vi "Get Section Names.vi"(8 "error in (no error)":errorcluster, 11 "Config in":refnum<class "LabVIEW-Config.lvclass">) -> (0 "error out":errorcluster, 1 "Section Names":string[](array[string]), 3 "Config out":refnum<class "LabVIEW-Config.lvclass">)   [LabVIEW 2017, in "LabVIEW-Config.lvlib" / "LabVIEW-Config.lvclass"]
uses:
  LabVIEW-Config.lvclass
  LabVIEW-Config.lvclass/LabVIEW-Config.ctl
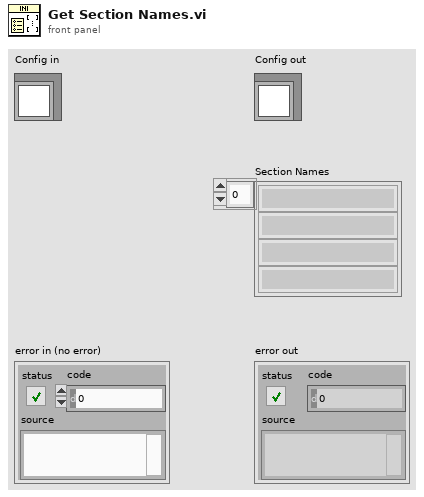
[diagram p1: front panel]
types:
  T1 = typedef "LabVIEW-Config.lvlib/LabVIEW-Config.lvclass/LineToken.ctl" = enum8{"comment", "section", "key", "more"}
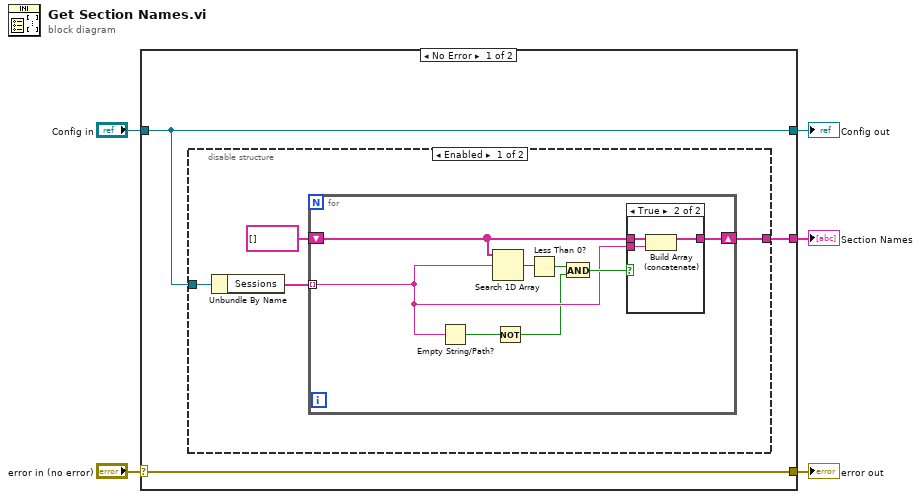
[diagram p0: block diagram]
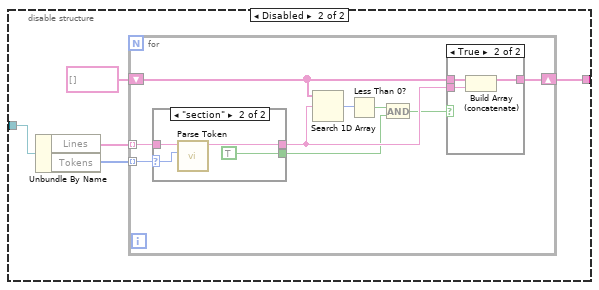
[diagram p3: hidden frame]
diagram:
  n1 = case shown="No Error" "error in (no error)" {
    selector: "error in (no error)" -> [w8 w48]
    tunnel: "Config in" -> [w7 w47]
    tunnel: [w6 _] -> w4
    tunnel: [w8 w48] -> w3
    tunnel: [w7 w47] -> w1
    frame No Error {
      n2 = disable-structure shown="Enabled" {
        disable-tunnel: w7 -> [w11 w27]
        disable-tunnel: [w9 w25] -> w6
        frame Enabled {
          n3 = Unbundle By Name(w11) -> ("Sessions"=w12:string[])
          n4 = for {
            tunnel: w12 -> [w15] mode=indexing
            shift-right: [w20] -> w9
            shift-left: string[] [] -> [w19]
            n5 = Empty String/Path?(string/path=w15) -> (empty?=w14:bool)
            n6 = Search 1D Array(1D array=w19, element=w15) -> (index of element=w18:i32)  [unwired: 1 in]
            n7 = Not(x=w14) -> (.not. x?=w13:bool)
            n8 = Less Than 0?(x=w18) -> (x < 0?=w17:bool)
            n9 = And(x=w17, y=w13) -> (x .and. y?=w16:bool)
            n10 = case shown="True" w16 {
              tunnel: [w21 w24] -> w20
              tunnel: w19 -> [w21 w23]
              tunnel: w15 -> [_ w22]
              frame False {
              }
              frame True {
                n11 = Build Array (concatenate)(w23, w22) -> (w24:string[])
              }
            }
          }
        }
        frame Disabled {
          n12 = Unbundle By Name(w27) -> ("Lines"=w28:string[], "Tokens"=w29:T1[])
          n13 = for {
            tunnel: w29 -> [w38] mode=indexing
            tunnel: w28 -> [w37] mode=indexing
            shift-right: [w36] -> w25
            shift-left: string[] [] -> [w35]
            n14 = case shown="\"section\"" w38 {
              selector: w38 -> [_ w44]
              tunnel: w37 -> [_ w45]
              tunnel: [_ w43] -> w34
              tunnel: [_ TRUE] -> w31
              frame Default {
              }
              frame "section" {
                n15 = call "Parse Token.vi"("Token"=w44, "Line"=w45) -> ("Name"=w43:string)  [unwired: 8 in, 1 out]
              }
            }
            n16 = Search 1D Array(1D array=w35, element=w34) -> (index of element=w33:i32)  [unwired: 1 in]
            n17 = Less Than 0?(x=w33) -> (x < 0?=w32:bool)
            n18 = And(x=w32, y=w31) -> (x .and. y?=w30:bool)
            n19 = case shown="True" w30 {
              tunnel: [w39 w42] -> w36
              tunnel: w35 -> [w39 w41]
              tunnel: w34 -> [_ w40]
              frame False {
              }
              frame True {
                n20 = Build Array (concatenate)(w41, w40) -> (w42:string[])
              }
            }
          }
        }
      }
    }
    frame Error {
    }
  }
  "error out" <- w3
  "Config out" <- w1
  "Section Names" <- w4
